vi "Rotork_Valve.vi"() -> ()   [LabVIEW 2014]
uses:
  <vilib>/rvi/Emulation/niFpgaGetClockAttributes.vi
  <vilib>/rvi/Emulation/niFpgaSctlEmulationGetInTimedLoop.vi
  <vilib>/rvi/Emulation/niFpgaEmulationReportErrorSimple.vi
  <vilib>/rvi/Emulation/niFpgaCriticalErrorInLSC.vi
panel:
  out "Valve position New":u8[](array[numeric])
  out "Valve position Old":u8[](array[numeric])
  out "valve 2":u8[](array[numeric])
  in  "Valve Array Out":u8[](array[numeric])=[65, 48, 48, 48, 48, 48, 13, 66, 48, 48, 48, 48, 48, 13, 67, 48, 48, 48, 48, 48, 13, 68, 48, 48, 48, 48, 48, 13, 73, 48, 48, 48, 48, 48, 13, 74, 48, 48, 48, 48, 48, 13, 75, 48, 48, 48, 48, 48, 13, 77, 48, 48, 48, 48, 48, 13, 0, 0, 0, 0]
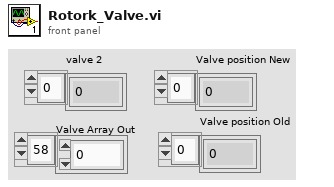
[diagram p1: front panel]
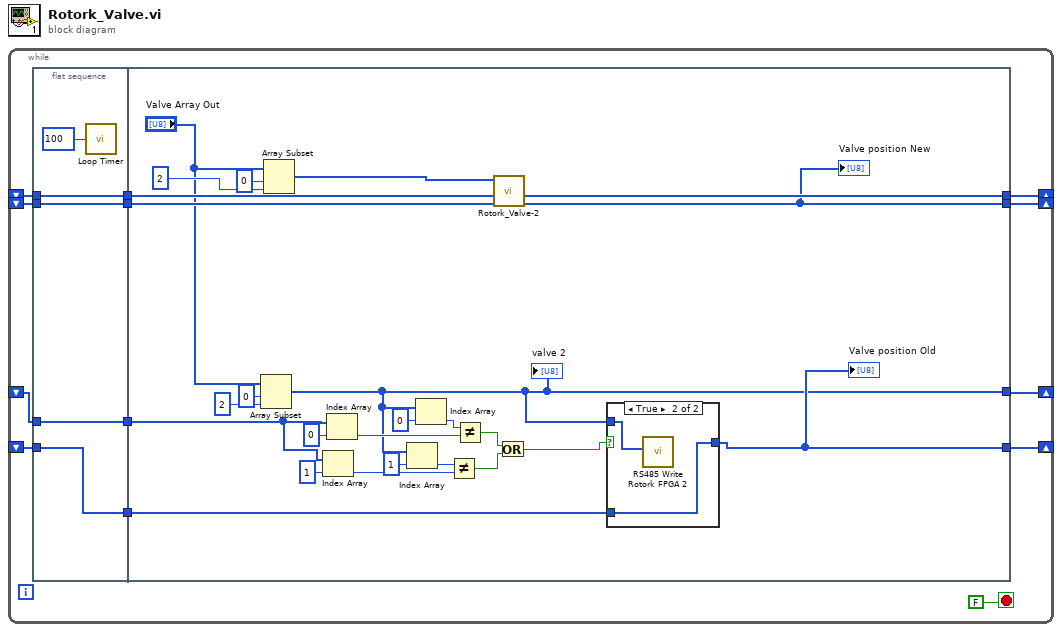
[diagram p0: block diagram]
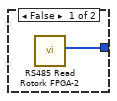
[diagram p2: hidden frame]
diagram:
  n1 = while {
    shift-right: [w12] -> _
    shift-left: _ -> [w10]
    shift-right: [w8] -> _
    shift-left: _ -> [w7]
    shift-right: [w6] -> _
    shift-left: _ -> [w2]
    shift-right: [w5] -> _
    shift-left: _ -> [w1]
    stop <- FALSE stop-if-true
    n2 = flat-sequence {
      tunnel: [w17] -> w11
      tunnel: w10 -> [w17]
      tunnel: w7 -> [w16]
      tunnel: [w16] -> w9
      tunnel: w2 -> [w15]
      tunnel: [w15] -> w4
      tunnel: w1 -> [w14]
      tunnel: [w14] -> w3
      tunnel: [w28] -> w12
      tunnel: w11 -> [w43]
      tunnel: w9 -> [w29]
      tunnel: [w27] -> w8
      tunnel: [w26] -> w6
      tunnel: [w19] -> w5
      tunnel: w4 -> [w25]
      tunnel: w3 -> [w24]
      frame #0 {
        n3 = call "Loop Timer"("Count(mSec)"=u32 100) -> ()  [unwired: 1 out]
      }
      frame #1 {
        n4 = Array Subset(array="Valve Array Out", index=0, length=2) -> (w27:u8[])
        "valve 2" <- w27
        n5 = Array Subset(array="Valve Array Out", index=0, length=2) -> (w23:u8[])
        n6 = Index Array(array=w29, index=1) -> (element=w40:u8)
        n7 = Index Array(array=w29, index=0) -> (element=w36:u8)
        n8 = Index Array(array=w27, index=1) -> (element=w42:u8)
        n9 = Index Array(array=w27, index=0) -> (element=w35:u8)
        n10 = Not Equal?(x=w42, y=w40) -> (x != y?=w39:bool)
        n11 = Not Equal?(x=w35, y=w36) -> (x != y?=w37:bool)
        n12 = call "Rotork_Valve-2.vi"("Array In 2"=w24, "Array In 1"=w25, "Valve SP"=w23) -> ("Array Out 2"=w19:u8[], "Array Out 1"=w26:u8[])  [unwired: 7 in]
        "Valve position New" <- w19
        n13 = Or(x=w37, y=w39) -> (x .or. y?=w32:bool)
        n14 = case shown="True" w32 {
          tunnel: [w44 w46] -> w28
          tunnel: w43 -> [_ w46]
          tunnel: w27 -> [_ w45]
          frame False {
            n15 = call "RS485 Read Rotork FPGA-2.vi"() -> ("Valve position"=w44:u8[])  [unwired: 11 in]
          }
          frame True {
            n16 = call "RS485 Write Rotork FPGA 2.vi"("Valve SP"=w45) -> ()  [unwired: 11 in]
          }
        }
        "Valve position Old" <- w28
      }
    }
  }
